vi "Create All Message Queues.vi"(8 "error in (no error)":errorcluster) -> (0 "error out":errorcluster, 3 "Message Queues out":T1)   [LabVIEW 2015, in "regser Message Queue.lvlib"]
doc: "This VI creates and initializes all the message queues for your application. If your application requires more than one message queue, right-click the \"Message Queues\" constant above and select Open Type Def. Add the new Message Queue(s) to the type definition, then initialize them in this VI."
uses:
  regser Message Queue.lvlib
  All Message Queues.ctl
  Message Cluster.ctl
  Enqueue Message (Array).vi
  Enqueue Message (Single).vi
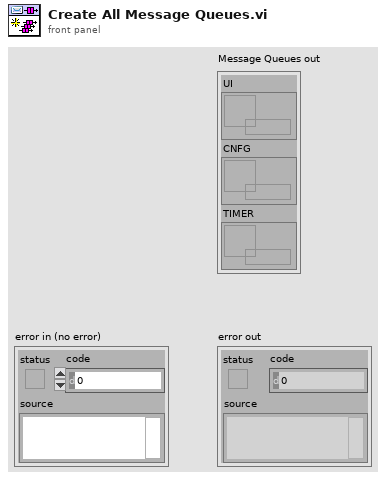
[diagram p1: front panel]
types:
  T1 = typedef "regser Message Queue.lvlib/All Message Queues.ctl" = cluster{"UI":refnum<queue>, "CNFG":refnum<queue>, "TIMER":refnum<queue>}
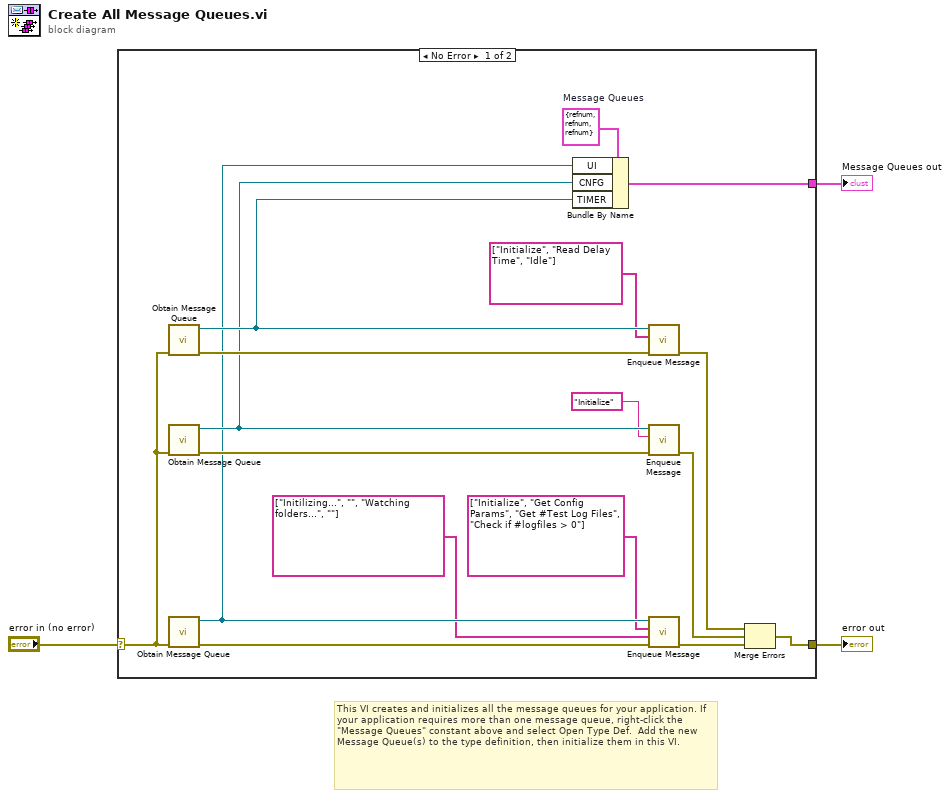
[diagram p0: block diagram]
diagram:
  # "This VI creates and initializes all the message queues for your application. If your application requires more than one message queue, right-click the \"Message Queues\" constant above and select Open Type Def.  Add the new Message Queue(s) to the type definition, then initialize them in this VI."
  n1 = case shown="No Error" "error in (no error)" {
    selector: "error in (no error)" -> [w13 w21]
    tunnel: [w15 w21] -> w3
    tunnel: [w17 _] -> w2
    frame No Error {
      w18 = T1 {"UI"=refnum, "CNFG"=refnum, "TIMER"=refnum}  # Message Queues
      n2 = call "Obtain Message Queue.vi"("error in (no error)"=w13) -> ("error out"=w12:errorcluster, "Message Queue"=w10:refnum<queue>)  [unwired: 9 in]
      n3 = call "Obtain Message Queue.vi"("error in (no error)"=w13) -> ("error out"=w20:errorcluster, "Message Queue"=w9:refnum<queue>)  [unwired: 9 in]
      n4 = call "Obtain Message Queue.vi"("error in (no error)"=w13) -> ("error out"=w16:errorcluster, "Message Queue"=w8:refnum<queue>)  [unwired: 9 in]
      n5 = Bundle By Name(cluster=w18, "UI"=w8, "CNFG"=w9, "TIMER"=w10) -> (w17:T1)
      n6 = call-poly "Enqueue Message.vi"("error in (no error)"=w12, "Message Array"=string[] ["Initialize", "Read Delay Time", "Idle"], "Message Queue"=w10) -> ("error out"=w11:errorcluster)  [unwired: 7 in, 1 out]
      n7 = call-poly "Enqueue Message.vi"("error in (no error)"=w20, "Message"="Initialize", "Message Queue"=w9) -> ("error out"=w14:errorcluster)  [unwired: 7 in, 1 out]
      n8 = call-poly "Enqueue Message.vi"("error in (no error)"=w16, "Message Data Array"=string[] ["Initilizing...", "", "Watching folders...", ""], "Message Array"=string[] ["Initialize", "Get Config Params", "Get #Test Log Files", "Check if #logfiles > 0"], "Message Queue"=w8) -> ("error out"=w19:errorcluster)  [unwired: 6 in, 1 out]
      n9 = Merge Errors(w11, w14, w19) -> (w15:errorcluster)
    }
    frame Error {
    }
  }
  "Message Queues out" <- w2
  "error out" <- w3
